vi "midioutshortmsg.vi"(4 "error in (no error)":errorcluster, 6 "data":i32 format="%.0x", 7 "MIDI output handle":i32) -> (0 "error out":errorcluster, 2 "Win32 error code":i32, 3 "duplicate MIDI output handle":i32)   [LabVIEW 2014]
doc: "Sends the MIDI keyboard information to the MIDI Output Device."
uses:
  winmm.dll
panel:
  # "Input Data"
  # "Local Data"
  # "Output Data"
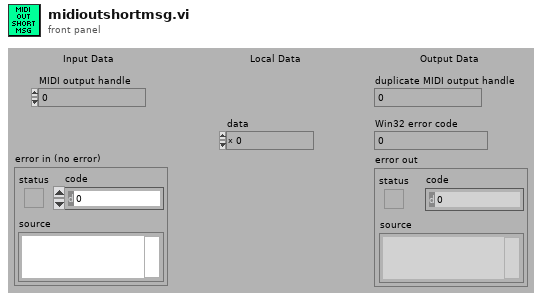
[diagram p1: front panel]
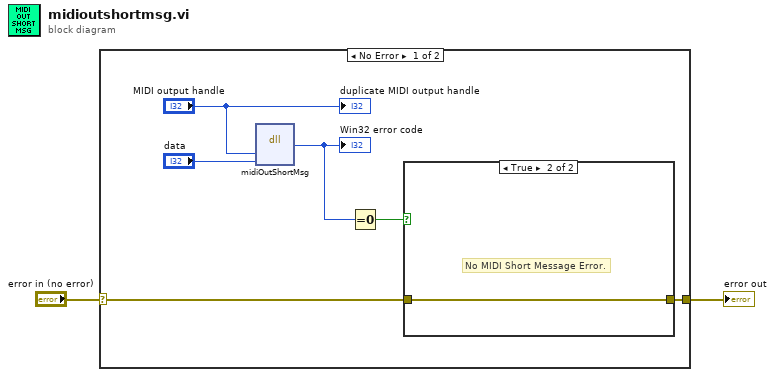
[diagram p0: block diagram]
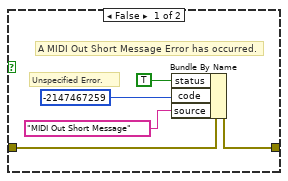
[diagram p2: hidden frame]
diagram:
  n1 = case shown="No Error" "error in (no error)" {
    selector: "error in (no error)" -> [w6 w15]
    tunnel: [w5 w15] -> w1
    frame No Error {
      n2 = dll-call lib="winmm.dll" fn="midiOutShortMsg"("hmidiout"="MIDI output handle", "data"="data") -> (w3:i32)  [unwired: 5 in, 2 out]
      "Win32 error code" <- w3
      n3 = Equal To 0?(x=w3) -> (x = 0?=w4:bool)
      n4 = case shown="True" w4 {
        tunnel: w6 -> [w13 w14]
        tunnel: [w12 w14] -> w5
        frame False {
          # "A MIDI Out Short Message Error has occurred."
          # "Unspecified Error."
          n5 = Bundle By Name(cluster=w13, "status"=TRUE, "code"=-2147467259, "source"="MIDI Out Short Message") -> (w12:errorcluster)
        }
        frame True {
          # "No MIDI Short Message Error."
        }
      }
      "duplicate MIDI output handle" <- "MIDI output handle"
    }
    frame Error {
    }
  }
  "error out" <- w1
